vi "read cluster.vi"(8 "error in (no error)":errorcluster, 9 "data value reference":refnum<data-value>, 10 "Tape Cluster":T1, 11 "controller in":refnum<class "controller.lvclass">) -> (0 "error out":errorcluster, 3 "controller out":refnum<class "controller.lvclass">)   [LabVIEW 2025, in "controller.lvclass"]
uses:
  controller.lvclass
  controller.lvclass/controller.ctl
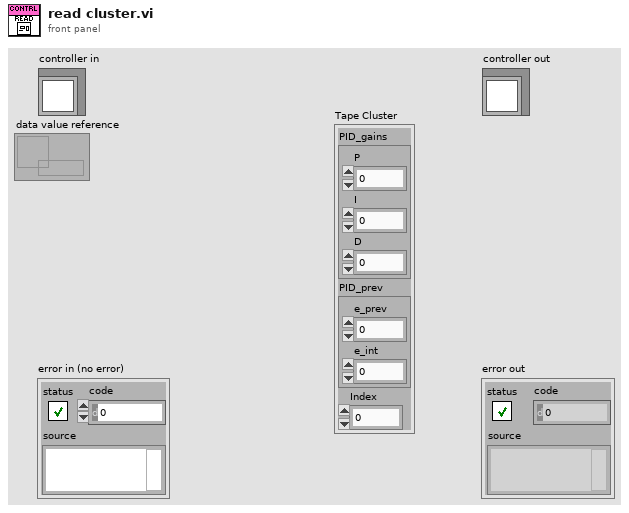
[diagram p1: front panel]
types:
  T1 = cluster{"PID_gains":cluster{"P":dbl, "I":dbl, "D":dbl}, "PID_prev":cluster{"e_prev":dbl, "e_int":dbl}, "Index":u32}
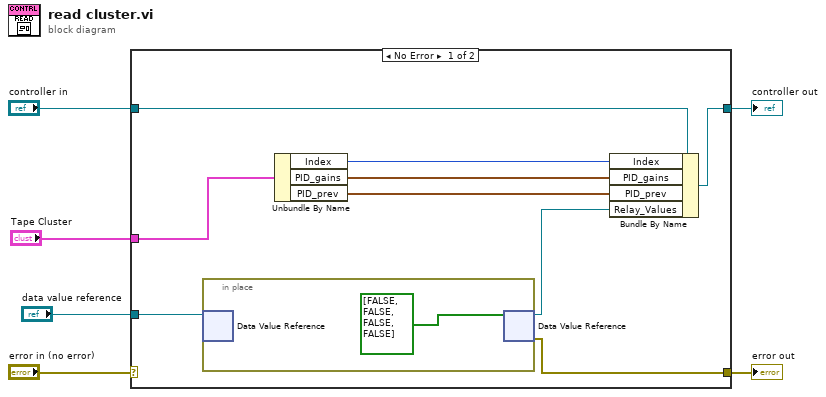
[diagram p0: block diagram]
diagram:
  n1 = case shown="No Error" "error in (no error)" {
    selector: "error in (no error)" -> [_ w18]
    tunnel: [w8 w18] -> w5
    tunnel: [w11 w17] -> w3
    tunnel: "controller in" -> [w12 w17]
    tunnel: "Tape Cluster" -> [w13 _]
    tunnel: "data value reference" -> [w10 _]
    frame No Error {
      n2 = in-place {
        n3 = in-place-dvr #1(w10) -> ()  [unwired: 2 out]
        n4 = in-place-dvr #1(bool[] [FALSE, FALSE, FALSE, FALSE] ("data")) -> (w9:refnum<data-value>, w8:errorcluster)
      }
      n5 = Unbundle By Name(w13) -> ("Index"=w7:u32, "PID_gains"=w14:cluster{"P":dbl, "I":dbl, "D":dbl}, "PID_prev"=w15:cluster{"e_prev":dbl, "e_int":dbl})
      n6 = Bundle By Name(cluster=w12, "Index"=w7, "PID_gains"=w14, "PID_prev"=w15, "Relay_Values"=w9) -> (w11:refnum<class "controller.lvclass">)
    }
    frame Error {
    }
  }
  "error out" <- w5
  "controller out" <- w3
